vi "Multidimensional Arrays.vi"() -> ()   [LabVIEW 2020]
panel:
  in  "3D Array":dbl[][][](array[numeric])
  in  "2D Array":dbl[][](array[numeric])
  in  "1D Array":dbl[](array[numeric])
  out "Scaler":dbl
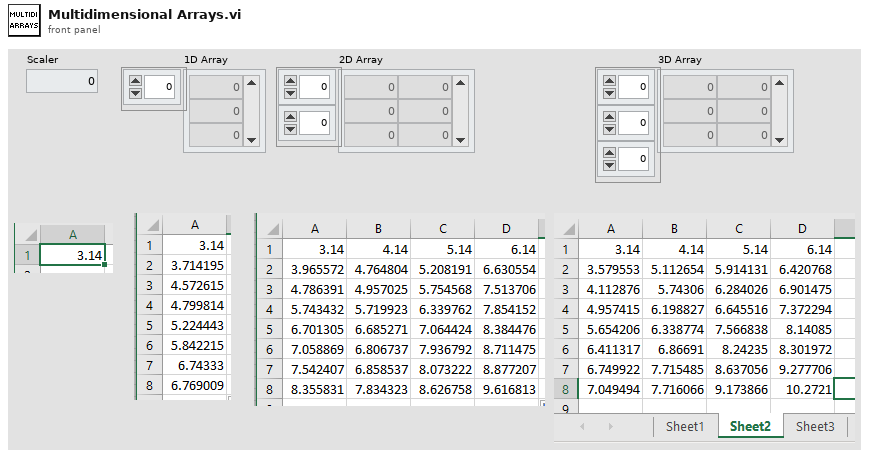
[diagram p1: front panel]
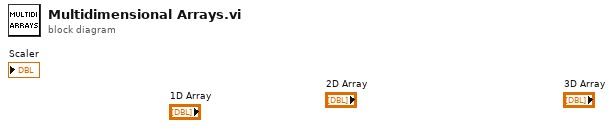
[diagram p0: block diagram]
diagram:
